vi "Test of Remove and Set-by-Names-Array Functions.vi"() -> ()   [LabVIEW 2011]
uses:
  JSON Object/JSON Object.lvclass
  JSON Object/Set Object Item by name.vi
  JSON Value/Set sub-Item by names.vi
  JSON Value/Get as JSON string (pretty).vi
  JSON Scalar/Set String.vi
  JSON Value/Remove sub-Item by names.vi
  JSON Scalar/Set Timestamp.vi
  JSON Scalar/Set DBL.vi
  JSON Array/Set JSON Array.vi
  JSON Value/Set Item by name array.vi
  JSON Scalar/JSON Scalar.lvclass
  Get Polymorphic/JSON GetSet.lvlib
  JSON Array/JSON Array.lvclass
  JSON Value/JSON Value.lvclass
panel:
  out "error out":errorcluster
  out "Final JSON String":string
  in  "Delete Path":string[](array[string])=["subObject", "DateTime"]
  out "Resulting JSON String":string
  in  "Replace Value (type: String)":string="Some Other Value"
  in  "Replace Path":string[](array[string])=["subObject", "String"]
  out "Generated JSON String":string
  # "Replace Path (case sensitive)\nThe path to the value object to insert or overwrite.\nSpecifying a path to an existing object overwrites it with the wired object\nSpecifying a non existing path inserts the wired object at that location,\nunless the path is inside a non-existing object - in which case the insert is\nskipped!\n\nLeaving the path empty also skips the insert..\n\nHere we replace the String value \"string\" in the subObject value object:"
  # "Delete Path (case sensitive)\nThe path to the value object to delete from the value object hierarchy.\nSpecifying a non existing path, or leaving the path empty skips the delete..\n\nHere we delete the TimeStamp value \"DateTime\" in the subObject value object:"
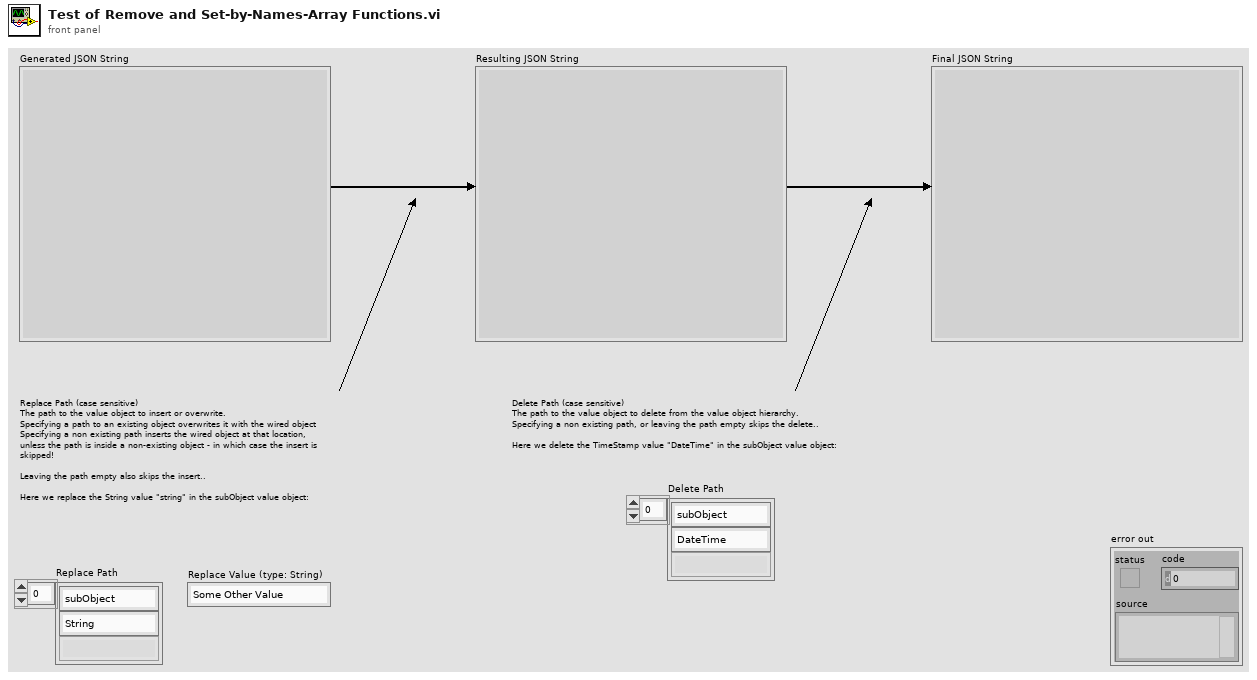
[diagram p1: front panel]
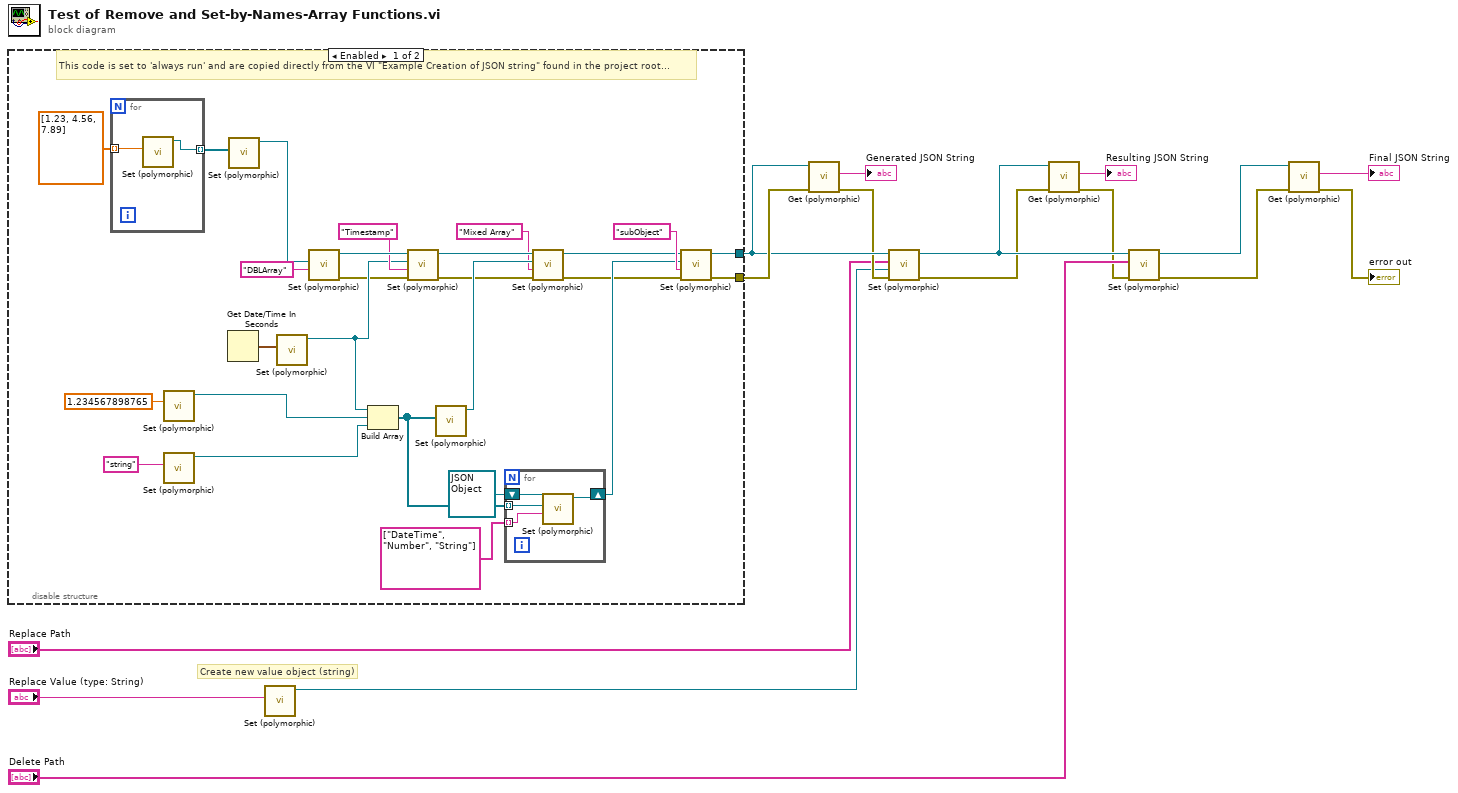
[diagram p0: block diagram]
diagram:
  # "Create new value object (string)"
  n1 = disable-structure shown="Enabled" {
    disable-tunnel: [w18 _] -> w14
    disable-tunnel: [w17 _] -> w16
    frame Enabled {
      # "This code is set to 'always run' and are copied directly from the VI \"Example Creation of JSON string\" found in the project root..."
      n2 = for {
        tunnel: dbl[] [1.23, 4.56, 7.89] -> [w48] mode=indexing
        tunnel: [w47] -> w41 mode=indexing
        n3 = call-poly "Set (polymorphic).vi"("Numeric"=w48) -> ("JSON Scalar out"=w47:refnum<class "JSON Scalar.lvclass">)  [unwired: 9 in, 1 out]
      }
      n4 = call-poly "Set (polymorphic).vi"("Numeric"=1.234567898765) -> ("JSON Scalar out"=w32:refnum<class "JSON Scalar.lvclass">)  [unwired: 9 in, 1 out]
      n5 = call-poly "Set (polymorphic).vi"("String"="string") -> ("JSON Scalar out"=w31:refnum<class "JSON Scalar.lvclass">)  [unwired: 9 in, 1 out]
      n6 = Get Date/Time In Seconds() -> (seconds since 1Jan1904=w37:timestamp)
      n7 = call-poly "Set (polymorphic).vi"("Array"=w41) -> ("JSON Array out"=w40:refnum<class "JSON Array.lvclass">)  [unwired: 9 in, 1 out]
      n8 = call-poly "Set (polymorphic).vi"("Time Stamp"=w37) -> ("JSON Scalar out"=w33:refnum<class "JSON Scalar.lvclass">)  [unwired: 9 in, 1 out]
      n9 = call-poly "Set (polymorphic).vi"("name"="DBLArray", "Value"=w40) -> ("error out"=w26:errorcluster, "JSON Object out"=w38:refnum<class "JSON Object.lvclass">)  [unwired: 7 in, 1 out]
      n10 = Build Array(w33, w32, w31) -> (w25:refnum<class "JSON Scalar.lvclass">[])
      n11 = call-poly "Set (polymorphic).vi"("error in (no error)"=w26, "name"="Timestamp", "Value"=w33, "JSON Object in"=w38) -> ("error out"=w27:errorcluster, "JSON Object out"=w30:refnum<class "JSON Object.lvclass">)  [unwired: 5 in, 1 out]
      n12 = call-poly "Set (polymorphic).vi"("Array"=w25) -> ("JSON Array out"=w29:refnum<class "JSON Array.lvclass">)  [unwired: 9 in, 1 out]
      n13 = for {
        tunnel: w25 -> [w46] mode=indexing
        shift-right: [w44] -> w20
        shift-left: refnum<class "JSON Object.lvclass"> refnum ("JSON Object out") -> [w45]
        tunnel: string[] ["DateTime", "Number", "String"] -> [w43] mode=indexing
        n14 = call-poly "Set (polymorphic).vi"("name"=w43, "Value"=w46, "JSON Object in"=w45) -> ("JSON Object out"=w44:refnum<class "JSON Object.lvclass">)  [unwired: 6 in, 2 out]
      }
      n15 = call-poly "Set (polymorphic).vi"("error in (no error)"=w27, "name"="Mixed Array", "Value"=w29, "JSON Object in"=w30) -> ("error out"=w19:errorcluster, "JSON Object out"=w21:refnum<class "JSON Object.lvclass">)  [unwired: 5 in, 1 out]
      n16 = call-poly "Set (polymorphic).vi"("error in (no error)"=w19, "name"="subObject", "Value"=w20, "JSON Object in"=w21) -> ("error out"=w17:errorcluster, "JSON Object out"=w18:refnum<class "JSON Object.lvclass">)  [unwired: 5 in, 1 out]
    }
    frame Disabled {
    }
  }
  n17 = call-poly "Set (polymorphic).vi"("String"="Replace Value (type: String)") -> ("JSON Scalar out"=w10:refnum<class "JSON Scalar.lvclass">)  [unwired: 9 in, 1 out]
  n18 = call-poly "Get (polymorphic).vi"("error in (no error)"=w16, "JSON Value in"=w14) -> ("error out"=w13:errorcluster, "String"=→"Generated JSON String":string)  [unwired: 8 in]
  n19 = call-poly "Set (polymorphic).vi"("error in (no error)"=w13, "Value"=w10, "Name Array"="Replace Path", "JSON Value In"=w14) -> ("error out"=w7:errorcluster, "JSON Value Out"=w8:refnum<class "JSON Object.lvclass">)  [unwired: 5 in, 1 out]
  n20 = call-poly "Get (polymorphic).vi"("error in (no error)"=w7, "JSON Value in"=w8) -> ("error out"=w5:errorcluster, "String"=→"Resulting JSON String":string)  [unwired: 8 in]
  n21 = call-poly "Set (polymorphic).vi"("error in (no error)"=w5, "Name Array"="Delete Path", "JSON Value In"=w8) -> ("error out"=w2:errorcluster, "JSON Value Out"=w3:refnum<class "JSON Object.lvclass">)  [unwired: 6 in, 1 out]
  n22 = call-poly "Get (polymorphic).vi"("error in (no error)"=w2, "JSON Value in"=w3) -> ("error out"=→"error out":errorcluster, "String"=→"Final JSON String":string)  [unwired: 8 in]
